vi "LightsOnGlobal.vi"() -> ()   [LabVIEW 2019]
panel:
  in  "Lights On":bool
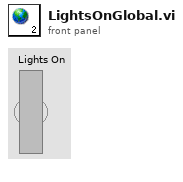
[diagram p1: front panel]
diagram:
